vi "RSZVB Get Internal Signal Source.vi"(8 "error in (no error)":errorcluster {"code" format="%.0x"}, 10 "Channel (1)":i32=1, 11 "VISA session":refnum<visa-resource-name>) -> (0 "error out":errorcluster {"code" format="%.0x"}, 2 "Internal Signal Source":i32, 3 "dup VISA session":refnum<visa-resource-name>)   [LabVIEW 2011]
doc: "This VI returns an analyzer port as a signal source for the LO signal (internal source).\n\nRemote-control command(s):\n[SENSe<Ch>:]FREQuency:CONVersion:MIXer:LOINternal?"
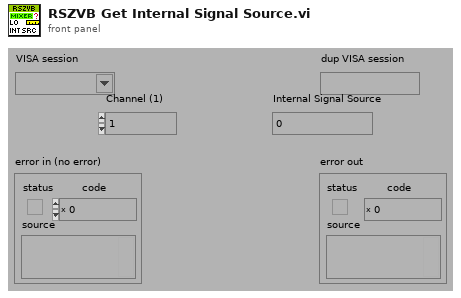
[diagram p1: front panel]
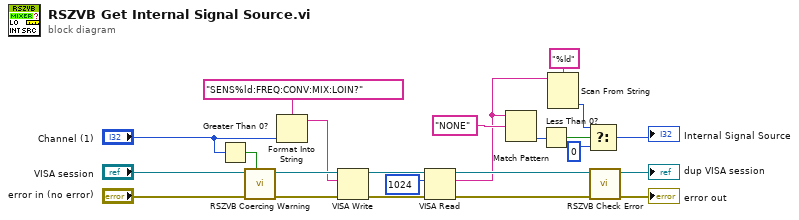
[diagram p0: block diagram]
diagram:
  n1 = Greater Than 0?(x="Channel (1)") -> (x > 0?=w21:bool)
  n2 = call "RSZVB Coercing Warning.vi"("In Range?"=w21, "error in (no error)"="error in (no error)", "VISA session"="VISA session") -> ("error out"=w22:errorcluster, "dup VISA session"=w23:refnum<visa-resource-name>)  [unwired: 7 in]
  n3 = Format Into String(format string="SENS%ld:FREQ:CONV:MIX:LOIN?", "Channel (1)") -> (resulting string=w14:string)  [unwired: 2 in, 1 out]
  n4 = VISA Write(VISA resource name=w23, write buffer=w14, error in (no error)=w22) -> (VISA resource name out=w18:refnum<visa-resource-name>, error out=w19:errorcluster)  [unwired: 1 out]
  n5 = VISA Read(VISA resource name=w18, byte count=u32 1024 ("byte count (0)"), error in (no error)=w19) -> (VISA resource name out=w16:refnum<visa-resource-name>, read buffer=w8:string, error out=w17:errorcluster)  [unwired: 1 out]
  n6 = Match Pattern(string=w8, regular expression="NONE") -> (offset past match=w12:i32)  [unwired: 1 in, 3 out]
  n7 = Less Than 0?(x=w12) -> (x < 0?=w11:bool)
  n8 = Scan From String(format string="%ld", input string=w8) -> (output 1=w7:i32)  [unwired: 3 in, 3 out]
  n9 = Select(t=w7, s=w11, f=0 ("byte count (0)")) -> (s? t:f=→"Internal Signal Source":i32)
  n10 = call "RSZVB Check Error.vi"("error in (no error)"=w17, "VISA session"=w16) -> ("error out"=→"error out":errorcluster, "dup VISA session"=→"dup VISA session":refnum<visa-resource-name>)  [unwired: 8 in]
